vi "诊断标定3.vi"(8 "CAN端口":u16(ring), 9 "设备索引号":u16(ring), 10 "CAN卡类型":u32(ring)=21) -> ()   [LabVIEW 2013] (continued)
            n1358 = property on="配置文件版本" class="Str"("Disabled"=w1841) -> ()  [unwired: 2 in, 2 out]
            n1359 = property on="项目信息" class="Tbl (严格)"("Disabled"=w1841) -> ()  [unwired: 2 in, 2 out]
            n1360 = property on="产品编号" class="Str"("Disabled"=w1841) -> ()  [unwired: 2 in, 2 out]
            n1361 = property on="车架(牌)号" class="Str"("Disabled"=w1841) -> ()  [unwired: 2 in, 2 out]
            n1362 = Select(t=0, s=w1833, f=1) -> (s? t:f=w1832:i32)
            n1363 = property on="项目信息2" class="Clust (严格)"("DisabledEnum"=w1832) -> ()  [unwired: 2 in, 2 out]
            n1364 = property on="SOH(%)" class="DigNum (严格)"("Disabled"=w1832) -> ()  [unwired: 2 in, 2 out]
            n1365 = global read "功能码全局.vi" "主板项目信息7"() -> (w1840:bool[])
            n1366 = Index Array(array=w1840, index #1=4 ("索引"), index #2=7 ("索引")) -> (element #1=w1837:bool, element #2=w1836:bool)
            n1367 = Not(x=w1843) -> (.not. x?=w1842:bool)
          }
          frame "SOC过低(2)", "SOC过高(2)", "SOH过低(2)", "充电电流过高(2)", "单体电压过低(2)", "单体电压过高(2)", "单组电压不均衡(2)", "单组温度不均衡(2)", "二级故障阀值", "放电电流过高(2)", "极柱温度过高(2)", "内阻过大(2)", "温度过低(2)", "温度过高(2)", "整组电压不均衡(2)", "整组温度不均衡(2)", "总电压过低(2)", "总电压过高(2)" {
            w1855 = FALSE
            n1368 = property on="从板个数" class="DigNum (严格)"("NumText.BGColor"=u32 13816530) -> ()  [unwired: 2 in, 2 out]
            n1369 = Select(t=0, s=w1847, f=1) -> (s? t:f=w1846:i32)
            n1370 = property on="一级故障 2" class="Clust (严格)"("DisabledEnum"=w1846) -> ()  [unwired: 2 in, 2 out]
            n1371 = global read "功能码全局.vi" "主板故障阀值9"() -> (w1853:bool[])
            n1372 = Index Array(array=w1853, index #1=3 ("索引"), index #2=6 ("索引")) -> (element #1=w1851:bool, element #2=w1850:bool)
            n1373 = Not(x=w1855) -> (.not. x?=w1856:bool)
          }
          frame "SOC过低(3)", "SOC过高(3)", "SOH过低(3)", "充电电流过高(3)", "单体电压过低(3)", "单体电压过高(3)", "单组电压不均衡(3)", "单组温度不均衡(3)", "放电电流过高(3)", "极柱温度过高(3)", "内阻过大(3)", "三级故障阀值", "温度过低(3)", "温度过高(3)", "整组电压不均衡(3)", "整组温度不均衡(3)", "总电压过低(3)", "总电压过高(3)" {
            w1869 = FALSE
            n1374 = property on="从板个数" class="DigNum (严格)"("NumText.BGColor"=u32 13816530) -> ()  [unwired: 2 in, 2 out]
            n1375 = Select(t=0, s=w1860, f=1) -> (s? t:f=w1859:i32)
            n1376 = property on="一级故障 3" class="Clust (严格)"("DisabledEnum"=w1859) -> ()  [unwired: 2 in, 2 out]
            n1377 = global read "功能码全局.vi" "主板故障阀值9"() -> (w1866:bool[])
            n1378 = Index Array(array=w1866, index #1=4 ("索引"), index #2=7 ("索引")) -> (element #1=w1864:bool, element #2=w1863:bool)
            n1379 = Not(x=w1869) -> (.not. x?=w1868:bool)
          }
          frame "SOC过低", "SOC过高", "SOH过低", "充电电流过高", "单体电压过低", "单体电压过高", "单组电压不均衡", "单组温度不均衡", "放电电流过高", "极柱温度过高", "内阻过大", "温度过低", "温度过高", "一级故障阀值", "整组电压不均衡", "整组温度不均衡", "总电压过低", "总电压过高" {
            w1882 = FALSE
            n1380 = Select(t=0, s=w1873, f=1) -> (s? t:f=w1872:i32)
            n1381 = property on="从板个数" class="DigNum (严格)"("NumText.BGColor"=u32 13816530) -> ()  [unwired: 2 in, 2 out]
            n1382 = property on="一级故障" class="Clust (严格)"("DisabledEnum"=w1872) -> ()  [unwired: 2 in, 2 out]
            n1383 = global read "功能码全局.vi" "主板故障阀值9"() -> (w1879:bool[])
            n1384 = Index Array(array=w1879, index #1=2 ("索引"), index #2=5 ("索引")) -> (element #1=w1877:bool, element #2=w1876:bool)
            n1385 = Not(x=w1882) -> (.not. x?=w1881:bool)
          }
          frame "充电控制参数", "电流步长", "最大允许充电电流", "最大允许充电温度", "最大允许单体电压", "最大允许总电压", "最小允许充电电流", "最小允许充电温度", "最小允许单体电压" {
            w1885 = 2
            w1896 = FALSE
            n1386 = property on="从板个数" class="DigNum (严格)"("NumText.BGColor"=u32 13816530) -> ()  [unwired: 2 in, 2 out]
            n1387 = property on="风机开启温度" class="DigNum (严格)"("Disabled"=w1885) -> ()  [unwired: 2 in, 2 out]
            n1388 = property on="风机关闭温度" class="DigNum (严格)"("Disabled"=w1885) -> ()  [unwired: 2 in, 2 out]
            n1389 = property on="加热开启温度" class="DigNum (严格)"("Disabled"=w1885) -> ()  [unwired: 2 in, 2 out]
            n1390 = property on="加热关闭温度" class="DigNum (严格)"("Disabled"=w1885) -> ()  [unwired: 2 in, 2 out]
            n1391 = property on="风机开启温差" class="DigNum (严格)"("Disabled"=w1885) -> ()  [unwired: 2 in, 2 out]
            n1392 = property on="风机关闭温差" class="DigNum (严格)"("Disabled"=w1885) -> ()  [unwired: 2 in, 2 out]
            n1393 = property on="加热控制参数" class="Clust (严格)"("DisabledEnum"=w1885) -> ()  [unwired: 2 in, 2 out]
            n1394 = Select(t=0, s=w1887, f=1) -> (s? t:f=w1886:i32)
            n1395 = property on="最大允许总电压" class="DigNum (严格)"("Disabled"=w1886) -> ()  [unwired: 2 in, 2 out]
            n1396 = property on="最大允许充电温度" class="DigNum (严格)"("Disabled"=w1886) -> ()  [unwired: 2 in, 2 out]
            n1397 = property on="最小允许充电温度" class="DigNum (严格)"("Disabled"=w1886) -> ()  [unwired: 2 in, 2 out]
            n1398 = property on="电流步长" class="DigNum (严格)"("Disabled"=w1886) -> ()  [unwired: 2 in, 2 out]
            n1399 = property on="最大允许单体电压" class="DigNum (严格)"("Disabled"=w1886) -> ()  [unwired: 2 in, 2 out]
            n1400 = property on="最小允许单体电压" class="DigNum (严格)"("Disabled"=w1886) -> ()  [unwired: 2 in, 2 out]
            n1401 = property on="最大允许充电电流" class="DigNum (严格)"("Disabled"=w1886) -> ()  [unwired: 2 in, 2 out]
            n1402 = property on="最小允许充电电流" class="DigNum (严格)"("Disabled"=w1886) -> ()  [unwired: 2 in, 2 out]
            n1403 = global read "功能码全局.vi" "主板控制类信息10"() -> (w1893:bool[])
            n1404 = Index Array(array=w1893, index #1=5 ("索引"), index #2=7 ("索引")) -> (element #1=w1891:bool, element #2=w1890:bool)
            n1405 = Not(x=w1896) -> (.not. x?=w1895:bool)
          }
          frame "风机关闭温差", "风机关闭温度", "风机开启温差", "风机开启温度", "加热关闭温差", "加热关闭温度", "加热开启温度", "加热控制参数" {
            w1908 = 2
            w1910 = FALSE
            n1406 = Select(t=0, s=w1900, f=1) -> (s? t:f=w1899:i32)
            n1407 = property on="从板个数" class="DigNum (严格)"("NumText.BGColor"=u32 13816530) -> ()  [unwired: 2 in, 2 out]
            n1408 = property on="加热控制参数" class="Clust (严格)"("DisabledEnum"=w1899) -> ()  [unwired: 2 in, 2 out]
            n1409 = property on="风机开启温度" class="DigNum (严格)"("Disabled"=w1899) -> ()  [unwired: 2 in, 2 out]
            n1410 = property on="风机关闭温度" class="DigNum (严格)"("Disabled"=w1899) -> ()  [unwired: 2 in, 2 out]
            n1411 = property on="加热开启温度" class="DigNum (严格)"("Disabled"=w1899) -> ()  [unwired: 2 in, 2 out]
            n1412 = property on="加热关闭温度" class="DigNum (严格)"("Disabled"=w1899) -> ()  [unwired: 2 in, 2 out]
            n1413 = property on="风机开启温差" class="DigNum (严格)"("Disabled"=w1899) -> ()  [unwired: 2 in, 2 out]
            n1414 = property on="风机关闭温差" class="DigNum (严格)"("Disabled"=w1899) -> ()  [unwired: 2 in, 2 out]
            n1415 = property on="最大允许总电压" class="DigNum (严格)"("Disabled"=w1908) -> ()  [unwired: 2 in, 2 out]
            n1416 = property on="最大允许充电温度" class="DigNum (严格)"("Disabled"=w1908) -> ()  [unwired: 2 in, 2 out]
            n1417 = property on="最小允许充电温度" class="DigNum (严格)"("Disabled"=w1908) -> ()  [unwired: 2 in, 2 out]
            n1418 = property on="电流步长" class="DigNum (严格)"("Disabled"=w1908) -> ()  [unwired: 2 in, 2 out]
            n1419 = property on="最大允许单体电压" class="DigNum (严格)"("Disabled"=w1908) -> ()  [unwired: 2 in, 2 out]
            n1420 = property on="最小允许单体电压" class="DigNum (严格)"("Disabled"=w1908) -> ()  [unwired: 2 in, 2 out]
            n1421 = property on="最大允许充电电流" class="DigNum (严格)"("Disabled"=w1908) -> ()  [unwired: 2 in, 2 out]
            n1422 = property on="最小允许充电电流" class="DigNum (严格)"("Disabled"=w1908) -> ()  [unwired: 2 in, 2 out]
            n1423 = global read "功能码全局.vi" "主板控制类信息10"() -> (w1906:bool[])
            n1424 = Index Array(array=w1906, index #1=4 ("索引"), index #2=6 ("索引")) -> (element #1=w1904:bool, element #2=w1903:bool)
            n1425 = Not(x=w1910) -> (.not. x?=w1909:bool)
          }
          frame "电池信息" {
            w1923 = FALSE
            n1426 = Select(t=0, s=w1914, f=1) -> (s? t:f=w1913:i32)
            n1427 = property on="电池串联" class="DigNum (严格)"("Disabled"=w1913) -> ()  [unwired: 2 in, 2 out]
            n1428 = property on="电池并联" class="DigNum (严格)"("Disabled"=w1913) -> ()  [unwired: 2 in, 2 out]
            n1429 = property on="电池包额定容量" class="DigNum (严格)"("Disabled"=w1913) -> ()  [unwired: 2 in, 2 out]
            n1430 = property on="电池包额定能量(kWh)" class="DigNum (严格)"("Disabled"=w1913) -> ()  [unwired: 2 in, 2 out]
            n1431 = property on="电池包额定总电压" class="DigNum (严格)"("Disabled"=w1913) -> ()  [unwired: 2 in, 2 out]
            n1432 = property on="实际容量" class="DigNum (严格)"("Disabled"=w1913) -> ()  [unwired: 2 in, 2 out]
            n1433 = property on="电池包组号" class="Str"("Disabled"=w1913) -> ()  [unwired: 2 in, 2 out]
            n1434 = property on="电池生产日期" class="Str"("Disabled"=w1913) -> ()  [unwired: 2 in, 2 out]
            n1435 = property on="电池厂家" class="Str"("Disabled"=w1913) -> ()  [unwired: 2 in, 2 out]
            n1436 = property on="电池类型" class="Str"("Disabled"=w1913) -> ()  [unwired: 2 in, 2 out]
            n1437 = property on="累计充电总安时" class="DigNum (严格)"("Disabled"=w1913) -> ()  [unwired: 2 in, 2 out]
            n1438 = property on="累计放电总安时" class="DigNum (严格)"("Disabled"=w1913) -> ()  [unwired: 2 in, 2 out]
            n1439 = property on="电池放空次数" class="DigNum (严格)"("Disabled"=w1913) -> ()  [unwired: 2 in, 2 out]
            n1440 = property on="电池充满次数" class="DigNum (严格)"("Disabled"=w1913) -> ()  [unwired: 2 in, 2 out]
            n1441 = property on="电池充电次数" class="DigNum (严格)"("Disabled"=w1913) -> ()  [unwired: 2 in, 2 out]
            n1442 = property on="电池信息" class="Clust (严格)"("DisabledEnum"=w1913) -> ()  [unwired: 2 in, 2 out]
            n1443 = global read "功能码全局.vi" "主板版本号11"() -> (w1920:bool[])
            n1444 = property on="从板个数" class="DigNum (严格)"("NumText.BGColor"=u32 13816530) -> ()  [unwired: 2 in, 2 out]
            n1445 = Index Array(array=w1920, index #1=0 ("索引"), index #2=1 ("索引")) -> (element #1=w1918:bool, element #2=w1917:bool)
            n1446 = Not(x=w1923) -> (.not. x?=w1922:bool)
          }
          frame "电池信息1" {
            w1935 = 2
            w1937 = FALSE
            n1447 = Select(t=0, s=w1927, f=1) -> (s? t:f=w1926:i32)
            n1448 = property on="电池信息" class="Clust (严格)"("DisabledEnum"=w1926) -> ()  [unwired: 2 in, 2 out]
            n1449 = property on="电池生产日期" class="Str"("Disabled"=w1926) -> ()  [unwired: 2 in, 2 out]
            n1450 = property on="电池厂家" class="Str"("Disabled"=w1926) -> ()  [unwired: 2 in, 2 out]
            n1451 = property on="电池类型" class="Str"("Disabled"=w1926) -> ()  [unwired: 2 in, 2 out]
            n1452 = property on="电池串联" class="DigNum (严格)"("Disabled"=w1926) -> ()  [unwired: 2 in, 2 out]
            n1453 = property on="电池并联" class="DigNum (严格)"("Disabled"=w1926) -> ()  [unwired: 2 in, 2 out]
            n1454 = property on="电池包额定容量" class="DigNum (严格)"("Disabled"=w1926) -> ()  [unwired: 2 in, 2 out]
            n1455 = property on="电池包额定能量(kWh)" class="DigNum (严格)"("Disabled"=w1926) -> ()  [unwired: 2 in, 2 out]
            n1456 = property on="电池包额定总电压" class="DigNum (严格)"("Disabled"=w1926) -> ()  [unwired: 2 in, 2 out]
            n1457 = property on="实际容量" class="DigNum (严格)"("Disabled"=w1926) -> ()  [unwired: 2 in, 2 out]
            n1458 = property on="累计充电总安时" class="DigNum (严格)"("Disabled"=w1935) -> ()  [unwired: 2 in, 2 out]
            n1459 = property on="累计放电总安时" class="DigNum (严格)"("Disabled"=w1935) -> ()  [unwired: 2 in, 2 out]
            n1460 = property on="电池放空次数" class="DigNum (严格)"("Disabled"=w1935) -> ()  [unwired: 2 in, 2 out]
            n1461 = property on="电池充满次数" class="DigNum (严格)"("Disabled"=w1935) -> ()  [unwired: 2 in, 2 out]
            n1462 = property on="电池充电次数" class="DigNum (严格)"("Disabled"=w1935) -> ()  [unwired: 2 in, 2 out]
            n1463 = property on="从板个数" class="DigNum (严格)"("NumText.BGColor"=u32 13816530) -> ()  [unwired: 2 in, 2 out]
            n1464 = property on="电池包组号" class="Str"("Disabled"=w1935) -> ()  [unwired: 2 in, 2 out]
            n1465 = global read "功能码全局.vi" "主板版本号11"() -> (w1933:bool[])
            n1466 = Index Array(array=w1933, index #1=0 ("索引"), index #2=1 ("索引")) -> (element #1=w1931:bool, element #2=w1930:bool)
            n1467 = Not(x=w1937) -> (.not. x?=w1936:bool)
          }
          frame "电池包组号" {
            w1949 = 2
            w1951 = FALSE
            n1468 = property on="电池生产日期" class="Str"("Disabled"=w1949) -> ()  [unwired: 2 in, 2 out]
            n1469 = property on="电池厂家" class="Str"("Disabled"=w1949) -> ()  [unwired: 2 in, 2 out]
            n1470 = property on="电池类型" class="Str"("Disabled"=w1949) -> ()  [unwired: 2 in, 2 out]
            n1471 = property on="电池串联" class="DigNum (严格)"("Disabled"=w1949) -> ()  [unwired: 2 in, 2 out]
            n1472 = property on="电池并联" class="DigNum (严格)"("Disabled"=w1949) -> ()  [unwired: 2 in, 2 out]
            n1473 = property on="电池包额定容量" class="DigNum (严格)"("Disabled"=w1949) -> ()  [unwired: 2 in, 2 out]
            n1474 = property on="电池包额定能量(kWh)" class="DigNum (严格)"("Disabled"=w1949) -> ()  [unwired: 2 in, 2 out]
            n1475 = property on="电池包额定总电压" class="DigNum (严格)"("Disabled"=w1949) -> ()  [unwired: 2 in, 2 out]
            n1476 = property on="实际容量" class="DigNum (严格)"("Disabled"=w1949) -> ()  [unwired: 2 in, 2 out]
            n1477 = property on="从板个数" class="DigNum (严格)"("NumText.BGColor"=u32 13816530) -> ()  [unwired: 2 in, 2 out]
            n1478 = property on="累计充电总安时" class="DigNum (严格)"("Disabled"=w1949) -> ()  [unwired: 2 in, 2 out]
            n1479 = property on="累计放电总安时" class="DigNum (严格)"("Disabled"=w1949) -> ()  [unwired: 2 in, 2 out]
            n1480 = property on="电池放空次数" class="DigNum (严格)"("Disabled"=w1949) -> ()  [unwired: 2 in, 2 out]
            n1481 = property on="电池充满次数" class="DigNum (严格)"("Disabled"=w1949) -> ()  [unwired: 2 in, 2 out]
            n1482 = property on="电池充电次数" class="DigNum (严格)"("Disabled"=w1949) -> ()  [unwired: 2 in, 2 out]
            n1483 = Select(t=0, s=w1941, f=1) -> (s? t:f=w1940:i32)
            n1484 = property on="电池包组号" class="Str"("Disabled"=w1940) -> ()  [unwired: 2 in, 2 out]
            n1485 = property on="电池信息" class="Clust (严格)"("DisabledEnum"=w1940) -> ()  [unwired: 2 in, 2 out]
            n1486 = global read "功能码全局.vi" "主板版本号11"() -> (w1947:bool[])
            n1487 = Index Array(array=w1947, index #1=0 ("索引"), index #2=1 ("索引")) -> (element #1=w1945:bool, element #2=w1944:bool)
            n1488 = Not(x=w1951) -> (.not. x?=w1950:bool)
          }
          frame "充放电安时" {
            w1963 = 2
            w1965 = FALSE
            n1489 = property on="电池生产日期" class="Str"("Disabled"=w1963) -> ()  [unwired: 2 in, 2 out]
            n1490 = property on="电池厂家" class="Str"("Disabled"=w1963) -> ()  [unwired: 2 in, 2 out]
            n1491 = property on="电池类型" class="Str"("Disabled"=w1963) -> ()  [unwired: 2 in, 2 out]
            n1492 = property on="电池串联" class="DigNum (严格)"("Disabled"=w1963) -> ()  [unwired: 2 in, 2 out]
            n1493 = property on="电池并联" class="DigNum (严格)"("Disabled"=w1963) -> ()  [unwired: 2 in, 2 out]
            n1494 = property on="电池包额定容量" class="DigNum (严格)"("Disabled"=w1963) -> ()  [unwired: 2 in, 2 out]
            n1495 = property on="电池包额定能量(kWh)" class="DigNum (严格)"("Disabled"=w1963) -> ()  [unwired: 2 in, 2 out]
            n1496 = property on="电池包额定总电压" class="DigNum (严格)"("Disabled"=w1963) -> ()  [unwired: 2 in, 2 out]
            n1497 = property on="实际容量" class="DigNum (严格)"("Disabled"=w1963) -> ()  [unwired: 2 in, 2 out]
            n1498 = property on="从板个数" class="DigNum (严格)"("NumText.BGColor"=u32 13816530) -> ()  [unwired: 2 in, 2 out]
            n1499 = Select(t=0, s=w1955, f=1) -> (s? t:f=w1954:i32)
            n1500 = property on="电池放空次数" class="DigNum (严格)"("Disabled"=w1963) -> ()  [unwired: 2 in, 2 out]
            n1501 = property on="电池充满次数" class="DigNum (严格)"("Disabled"=w1963) -> ()  [unwired: 2 in, 2 out]
            n1502 = property on="电池充电次数" class="DigNum (严格)"("Disabled"=w1963) -> ()  [unwired: 2 in, 2 out]
            n1503 = property on="电池包组号" class="Str"("Disabled"=w1963) -> ()  [unwired: 2 in, 2 out]
            n1504 = property on="累计充电总安时" class="DigNum (严格)"("Disabled"=w1954) -> ()  [unwired: 2 in, 2 out]
            n1505 = property on="累计放电总安时" class="DigNum (严格)"("Disabled"=w1954) -> ()  [unwired: 2 in, 2 out]
            n1506 = property on="电池信息" class="Clust (严格)"("DisabledEnum"=w1954) -> ()  [unwired: 2 in, 2 out]
            n1507 = global read "功能码全局.vi" "主板版本号11"() -> (w1961:bool[])
            n1508 = Index Array(array=w1961, index #1=0 ("索引"), index #2=1 ("索引")) -> (element #1=w1959:bool, element #2=w1958:bool)
            n1509 = Not(x=w1965) -> (.not. x?=w1964:bool)
          }
          frame "电池充放电次数" {
            w1977 = 2
            w1979 = FALSE
            n1510 = property on="从板个数" class="DigNum (严格)"("NumText.BGColor"=u32 13816530) -> ()  [unwired: 2 in, 2 out]
            n1511 = property on="电池生产日期" class="Str"("Disabled"=w1977) -> ()  [unwired: 2 in, 2 out]
            n1512 = property on="电池厂家" class="Str"("Disabled"=w1977) -> ()  [unwired: 2 in, 2 out]
            n1513 = property on="电池类型" class="Str"("Disabled"=w1977) -> ()  [unwired: 2 in, 2 out]
            n1514 = property on="电池串联" class="DigNum (严格)"("Disabled"=w1977) -> ()  [unwired: 2 in, 2 out]
            n1515 = property on="电池并联" class="DigNum (严格)"("Disabled"=w1977) -> ()  [unwired: 2 in, 2 out]
            n1516 = property on="电池包额定容量" class="DigNum (严格)"("Disabled"=w1977) -> ()  [unwired: 2 in, 2 out]
            n1517 = property on="电池包额定能量(kWh)" class="DigNum (严格)"("Disabled"=w1977) -> ()  [unwired: 2 in, 2 out]
            n1518 = property on="电池包额定总电压" class="DigNum (严格)"("Disabled"=w1977) -> ()  [unwired: 2 in, 2 out]
            n1519 = property on="实际容量" class="DigNum (严格)"("Disabled"=w1977) -> ()  [unwired: 2 in, 2 out]
            n1520 = Select(t=0, s=w1969, f=1) -> (s? t:f=w1968:i32)
            n1521 = property on="电池放空次数" class="DigNum (严格)"("Disabled"=w1968) -> ()  [unwired: 2 in, 2 out]
            n1522 = property on="电池充满次数" class="DigNum (严格)"("Disabled"=w1968) -> ()  [unwired: 2 in, 2 out]
            n1523 = property on="电池充电次数" class="DigNum (严格)"("Disabled"=w1968) -> ()  [unwired: 2 in, 2 out]
            n1524 = property on="累计充电总安时" class="DigNum (严格)"("Disabled"=w1977) -> ()  [unwired: 2 in, 2 out]
            n1525 = property on="累计放电总安时" class="DigNum (严格)"("Disabled"=w1977) -> ()  [unwired: 2 in, 2 out]
            n1526 = property on="电池信息" class="Clust (严格)"("DisabledEnum"=w1968) -> ()  [unwired: 2 in, 2 out]
            n1527 = property on="电池包组号" class="Str"("Disabled"=w1977) -> ()  [unwired: 2 in, 2 out]
            n1528 = global read "功能码全局.vi" "主板版本号11"() -> (w1975:bool[])
            n1529 = Index Array(array=w1975, index #1=0 ("索引"), index #2=1 ("索引")) -> (element #1=w1973:bool, element #2=w1972:bool)
            n1530 = Not(x=w1979) -> (.not. x?=w1978:bool)
          }
          frame "假", Default {
            w1984 = FALSE
            n1531 = Not(x=w1984) -> (.not. x?=w1983:bool)
          }
        }
        n1532 = property on="单个读取" class="Bool (严格)"("Visible"=w1452) -> ()  [unwired: 2 in, 2 out]
        n1533 = property on="单个写入" class="Bool (严格)"("Visible"=w1451) -> ()  [unwired: 2 in, 2 out]
        n1534 = local write "1"(w1459) -> ()
        n1535 = local write "1 2"(w1458) -> ()
        n1536 = local write "1 3"(w1457) -> ()
        n1537 = local write "1 4"(w1456) -> ()
        n1538 = local write "1 5"(w1455) -> ()
        n1539 = local write "1 11"(w1454) -> ()
        n1540 = local write "主板2"(w1460) -> ()
      }
      event "从板选项": Mouse Down {
        n1541 = event-data() -> ("CtlRef"=w1999:refnum<vi>)  [unwired: 8 out]
        n1542 = property class="Tree (严格)"(reference=w1999) -> ("Value"=w1998:string)  [unwired: 1 in, 2 out]
        n1543 = global read "功能码全局.vi" "主板监控2"() -> (w1989:bool[])
        n1544 = Index Array(array=w1989, index=6 ("索引")) -> (element=w1987:bool)
        n1545 = case shown="\"二维码\"" w1998 {
          tunnel: [T19."从板信息" ("等级 2") T19."从板信息" ("等级 2") T19."从板信息" ("等级 2") T19."从板信息" ("等级 2") T19."从板信息" ("等级 2") T19."从板信息" ("等级 2") T19."从板信息" ("等级 2") T19."从板信息" ("等级 2") T19."一级故障阀值" ("等级 2") T19."二级故障阀值" ("等级 2") T19."三级故障阀值" ("等级 2") T19."快换参数" ("等级 2") T19."快换参数" ("等级 2") T19."快换参数" ("等级 2") T19."快换参数" ("等级 2") T19."快换参数" ("等级 2") T19."快换参数" ("等级 2") T19."快换参数" ("等级 2") T19."快换参数" ("等级 2") T14."均衡参数" ("等级 2") T14."均衡参数" ("等级 2") T14."均衡参数" ("等级 2") T19."从板信息" ("等级 2")] -> w1997
          tunnel: [w2010 w2020 w2030 w2044 w2059 w2094 w2131 w2168 w2192 w2205 w2218 w2231 w2257 w2271 w2287 w2304 w2321 w2339 w2358 w2375 w2388 w2402 w2417] -> w1996
          tunnel: [w2002 w2012 w2022 w2032 w2046 w2081 w2118 w2155 w2203 w2205 w2218 w2231 w2257 w2271 w2287 w2304 w2321 w2339 w2358 w2375 w2388 w2402 w2416] -> w1995
          tunnel: [w2002 w2012 w2022 w2032 w2046 w2081 w2118 w2155 w2192 w2216 w2218 w2231 w2257 w2271 w2287 w2304 w2321 w2339 w2358 w2375 w2388 w2402 w2416] -> w1994
          tunnel: [w2002 w2012 w2022 w2032 w2046 w2081 w2118 w2155 w2192 w2205 w2229 w2231 w2257 w2271 w2287 w2304 w2321 w2339 w2358 w2375 w2388 w2402 w2416] -> w1993
          tunnel: [w2002 w2012 w2022 w2032 w2046 w2081 w2118 w2155 w2192 w2205 w2218 w2255 w2269 w2285 w2302 w2319 w2337 w2356 w2373 w2375 w2388 w2402 w2416] -> w1992
          tunnel: [w2007 w2017 w2023 w2039 w2053 w2088 w2125 w2162 w2199 w2212 w2225 w2240 w2262 w2277 w2291 w2309 w2324 w2344 w2362 w2378 w2392 w2407 w2416] -> w1991
          tunnel: [w2004 w2014 w2023 w2038 w2052 w2087 w2124 w2161 w2198 w2211 w2224 w2232 w2261 w2276 w2290 w2310 w2325 w2343 w2361 w2377 w2391 w2406 w2416] -> w1990
          tunnel: w1987 -> [_ _ w2027 w2035 w2049 w2084 w2121 w2158 w2194 w2208 w2221 w2252 w2265 w2280 w2295 w2313 w2329 w2347 w2366 w2381 w2395 w2409 _]
          tunnel: [w2002 w2012 w2022 w2032 w2046 w2081 w2118 w2155 w2192 w2205 w2218 w2231 w2257 w2271 w2287 w2304 w2321 w2339 w2358 w2376 w2389 w2403 w2416] -> w1986
          frame "从板号" {
            w2009 = 2
            w2002 = FALSE ("1 6")
            n1546 = property on="项目信息 2" class="Tbl (严格)"("Disabled"=w2009) -> ()  [unwired: 2 in, 2 out]
            n1547 = property on="加热控制参数" class="Clust (严格)"("Disabled"=w2009) -> ()  [unwired: 2 in, 2 out]
            n1548 = property on="从板号" class="DigNum (严格)"("NumText.BGColor"=u32 6618880) -> ()  [unwired: 2 in, 2 out]
            n1549 = global read "功能码全局.vi" "16"() -> (w2006:bool[])
            n1550 = Index Array(array=w2006, index #1=4 ("索引"), index #2=6 ("索引")) -> (element #1=w2007:bool, element #2=w2004:bool)
            n1551 = Not(x=w2002) -> (.not. x?=w2010:bool)
          }
          frame "二维码" {
            w2019 = 2
            w2012 = FALSE ("1 6")
            n1552 = property on="项目信息 2" class="Tbl (严格)"("Disabled"=w2019) -> ()  [unwired: 2 in, 2 out]
            n1553 = property on="加热控制参数" class="Clust (严格)"("Disabled"=w2019) -> ()  [unwired: 2 in, 2 out]
            n1554 = property on="从板号" class="DigNum (严格)"("NumText.BGColor"=u32 6618880) -> ()  [unwired: 2 in, 2 out]
            n1555 = global read "功能码全局.vi" "16"() -> (w2016:bool[])
            n1556 = Index Array(array=w2016, index #1=4 ("索引"), index #2=6 ("索引")) -> (element #1=w2017:bool, element #2=w2014:bool)
            n1557 = Not(x=w2012) -> (.not. x?=w2020:bool)
          }
          frame "从板信息" {
            w2022 = FALSE ("1 6")
            n1558 = Select(t=0, s=w2027, f=1) -> (s? t:f=w2026:i32)
            n1559 = property on="从板号" class="DigNum (严格)"("NumText.BGColor"=u32 16777215) -> ()  [unwired: 2 in, 2 out]
            n1560 = property on="项目信息 2" class="Tbl (严格)"("Disabled"=w2026) -> ()  [unwired: 2 in, 2 out]
            n1561 = property on="加热控制参数" class="Clust (严格)"("Disabled"=w2026) -> ()  [unwired: 2 in, 2 out]
            n1562 = Not(x=w2022) -> (.not. x?=w2030:bool)
            n1563 = local read "从板项目信息"() -> (w2024:bool)
            n1564 = Not(x=w2024) -> (.not. x?=w2023:bool)
          }
          frame "风机关闭温差", "风机关闭温度", "风机开启温差", "风机开启温度", "加热关闭温差", "加热关闭温度", "加热开启温度", "加热控制参数" {
            w2032 = FALSE ("1 6")
            n1565 = property on="从板号" class="DigNum (严格)"("NumText.BGColor"=u32 16777215) -> ()  [unwired: 2 in, 2 out]
            n1566 = Select(t=0, s=w2035, f=1) -> (s? t:f=w2034:i32)
            n1567 = property on="项目信息 2" class="Tbl (严格)"("Disabled"=2) -> ()  [unwired: 2 in, 2 out]
            n1568 = property on="加热控制参数" class="Clust (严格)"("Disabled"=w2034) -> ()  [unwired: 2 in, 2 out]
            n1569 = global read "功能码全局.vi" "16"() -> (w2041:bool[])
            n1570 = Index Array(array=w2041, index #1=5 ("索引"), index #2=7 ("索引")) -> (element #1=w2039:bool, element #2=w2038:bool)
            n1571 = Not(x=w2032) -> (.not. x?=w2044:bool)
          }
          frame "电压个数" {
            w2046 = FALSE ("1 6")
            n1572 = property on="从板号" class="DigNum (严格)"("NumText.BGColor"=u32 16777215) -> ()  [unwired: 2 in, 2 out]
            n1573 = control-ref of="项目信息 2"() -> (w2057:refnum<vi>)
            n1574 = stacked-sequence {
              tunnel: w2057 -> [w2064 w2066 w2075]
              frame #0 {
                n1575 = Bundle(0, 0) -> (w2063:cluster{i32, i32})  [unwired: 1 out]
                n1576 = property class="Tbl (严格)"(reference=w2064, "Index Values"=w2063) -> ()  [unwired: 1 in, 2 out]
              }
              frame #1 {
                n1577 = for {
                  N: 40 -> [_]
                  tunnel: w2066 -> [w2073]
                  i -> [w2068]
                  n1578 = Compound Arithmetic op=ADD(0 ("值"), w2068) -> (w2070:i32)
                  n1579 = Bundle(w2070, 0) -> (w2072:cluster{i32, i32})  [unwired: 1 out]
                  n1580 = property class="Tbl (严格)"(reference=w2073, "Active Cell"=w2072, "Cell BG Color"=u32 16448250) -> ()  [unwired: 1 in, 2 out]
                }
              }
              frame #2 {
                n1581 = for {
                  N: 1 -> [_]
                  tunnel: w2075 -> [w2080]
                  i -> [w2076]
                  n1582 = Bundle(w2076, 0) -> (w2079:cluster{i32, i32})  [unwired: 1 out]
                  n1583 = property class="Tbl (严格)"(reference=w2080, "Active Cell"=w2079, "Cell BG Color"=u32 6618880) -> ()  [unwired: 1 in, 2 out]
                }
              }
            }
            n1584 = Select(t=0, s=w2049, f=1) -> (s? t:f=w2048:i32)
            n1585 = property on="项目信息 2" class="Tbl (严格)"("Disabled"=w2048) -> ()  [unwired: 2 in, 2 out]
            n1586 = property on="加热控制参数" class="Clust (严格)"("Disabled"=2) -> ()  [unwired: 2 in, 2 out]
            n1587 = global read "功能码全局.vi" "15"() -> (w2055:bool[])
            n1588 = Index Array(array=w2055, index #1=0 ("索引"), index #2=4 ("索引")) -> (element #1=w2053:bool, element #2=w2052:bool)
            n1589 = Not(x=w2046) -> (.not. x?=w2059:bool)
          }
          frame "通道电压节数" {
            w2081 = FALSE ("1 6")
            n1590 = property on="从板号" class="DigNum (严格)"("NumText.BGColor"=u32 16777215) -> ()  [unwired: 2 in, 2 out]
            n1591 = control-ref of="项目信息 2"() -> (w2092:refnum<vi>)
            n1592 = stacked-sequence {
              tunnel: w2092 -> [w2099 w2101 w2110]
              frame #0 {
                n1593 = Bundle(22, 0) -> (w2098:cluster{i32, i32})  [unwired: 1 out]
                n1594 = property class="Tbl (严格)"(reference=w2099, "Index Values"=w2098) -> ()  [unwired: 1 in, 2 out]
              }
              frame #1 {
                n1595 = for {
                  N: 40 -> [_]
                  tunnel: w2101 -> [w2108]
                  i -> [w2103]
                  n1596 = Compound Arithmetic op=ADD(0 ("值"), w2103) -> (w2105:i32)
                  n1597 = Bundle(w2105, 0) -> (w2107:cluster{i32, i32})  [unwired: 1 out]
                  n1598 = property class="Tbl (严格)"(reference=w2108, "Active Cell"=w2107, "Cell BG Color"=u32 16448250) -> ()  [unwired: 1 in, 2 out]
                }
              }
              frame #2 {
                n1599 = for {
                  N: 5 -> [_]
                  tunnel: w2110 -> [w2117]
                  i -> [w2113]
                  n1600 = Add(x=22, y=w2113) -> (x+y=w2112:i32)
                  n1601 = Bundle(w2112, 0) -> (w2116:cluster{i32, i32})  [unwired: 1 out]
                  n1602 = property class="Tbl (严格)"(reference=w2117, "Active Cell"=w2116, "Cell BG Color"=u32 6618880) -> ()  [unwired: 1 in, 2 out]
                }
              }
            }
            n1603 = Select(t=0, s=w2084, f=1) -> (s? t:f=w2083:i32)
            n1604 = property on="项目信息 2" class="Tbl (严格)"("Disabled"=w2083) -> ()  [unwired: 2 in, 2 out]
            n1605 = property on="加热控制参数" class="Clust (严格)"("Disabled"=2) -> ()  [unwired: 2 in, 2 out]
            n1606 = global read "功能码全局.vi" "15"() -> (w2090:bool[])
            n1607 = Index Array(array=w2090, index #1=1 ("索引"), index #2=5 ("索引")) -> (element #1=w2088:bool, element #2=w2087:bool)
            n1608 = Not(x=w2081) -> (.not. x?=w2094:bool)
          }
          frame "保险位置" {
            w2118 = FALSE ("1 6")
            n1609 = control-ref of="项目信息 2"() -> (w2129:refnum<vi>)
            n1610 = stacked-sequence {
              tunnel: w2129 -> [w2136 w2138 w2147]
              frame #0 {
                n1611 = Bundle(0, 0) -> (w2135:cluster{i32, i32})  [unwired: 1 out]
                n1612 = property class="Tbl (严格)"(reference=w2136, "Index Values"=w2135) -> ()  [unwired: 1 in, 2 out]
              }
              frame #1 {
                n1613 = for {
                  N: 40 -> [_]
                  tunnel: w2138 -> [w2145]
                  i -> [w2141]
                  n1614 = Add(x=2, y=w2141) -> (x+y=w2140:i32)
                  n1615 = Bundle(w2140, 0) -> (w2144:cluster{i32, i32})  [unwired: 1 out]
                  n1616 = property class="Tbl (严格)"(reference=w2145, "Active Cell"=w2144, "Cell BG Color"=u32 16448250) -> ()  [unwired: 1 in, 2 out]
                }
              }
              frame #2 {
                n1617 = for {
                  N: 20 -> [_]
                  tunnel: w2147 -> [w2154]
                  i -> [w2150]
                  n1618 = Add(x=2, y=w2150) -> (x+y=w2149:i32)
                  n1619 = Bundle(w2149, 0) -> (w2153:cluster{i32, i32})  [unwired: 1 out]
                  n1620 = property class="Tbl (严格)"(reference=w2154, "Active Cell"=w2153, "Cell BG Color"=u32 6618880) -> ()  [unwired: 1 in, 2 out]
                }
              }
            }
            n1621 = property on="从板号" class="DigNum (严格)"("NumText.BGColor"=u32 16777215) -> ()  [unwired: 2 in, 2 out]
            n1622 = Select(t=0, s=w2121, f=1) -> (s? t:f=w2120:i32)
            n1623 = property on="项目信息 2" class="Tbl (严格)"("Disabled"=w2120) -> ()  [unwired: 2 in, 2 out]
            n1624 = property on="加热控制参数" class="Clust (严格)"("Disabled"=2) -> ()  [unwired: 2 in, 2 out]
            n1625 = global read "功能码全局.vi" "15"() -> (w2127:bool[])
            n1626 = Index Array(array=w2127, index #1=2 ("索引"), index #2=6 ("索引")) -> (element #1=w2125:bool, element #2=w2124:bool)
            n1627 = Not(x=w2118) -> (.not. x?=w2131:bool)
          }
          frame "温度个数" {
            w2155 = FALSE ("1 6")
            n1628 = control-ref of="项目信息 2"() -> (w2166:refnum<vi>)
            n1629 = stacked-sequence {
              tunnel: w2166 -> [w2173 w2174 w2184]
              frame #0 {
                n1630 = Bundle(0, 0) -> (w2172:cluster{i32, i32})  [unwired: 1 out]
                n1631 = property class="Tbl (严格)"(reference=w2173, "Index Values"=w2172) -> ()  [unwired: 1 in, 2 out]
              }
              frame #1 {
                n1632 = for {
                  N: 40 -> [_]
                  tunnel: w2174 -> [w2182]
                  i -> [w2177]
                  n1633 = Compound Arithmetic op=ADD(0 ("值"), w2177) -> (w2179:i32)
                  n1634 = Bundle(w2179, 0) -> (w2181:cluster{i32, i32})  [unwired: 1 out]
                  n1635 = property class="Tbl (严格)"(reference=w2182, "Active Cell"=w2181, "Cell BG Color"=u32 16448250) -> ()  [unwired: 1 in, 2 out]
                }
              }
              frame #2 {
                n1636 = for {
                  N: 1 -> [_]
                  tunnel: w2184 -> [w2191]
                  i -> [w2187]
                  n1637 = Add(x=1, y=w2187) -> (x+y=w2186:i32)
                  n1638 = Bundle(w2186, 0) -> (w2190:cluster{i32, i32})  [unwired: 1 out]
                  n1639 = property class="Tbl (严格)"(reference=w2191, "Active Cell"=w2190, "Cell BG Color"=u32 6618880) -> ()  [unwired: 1 in, 2 out]
                }
              }
            }
            n1640 = Select(t=0, s=w2158, f=1) -> (s? t:f=w2157:i32)
            n1641 = property on="项目信息 2" class="Tbl (严格)"("Disabled"=w2157) -> ()  [unwired: 2 in, 2 out]
            n1642 = property on="加热控制参数" class="Clust (严格)"("Disabled"=2) -> ()  [unwired: 2 in, 2 out]
            n1643 = property on="从板号" class="DigNum (严格)"("NumText.BGColor"=u32 16777215) -> ()  [unwired: 2 in, 2 out]
            n1644 = global read "功能码全局.vi" "15"() -> (w2164:bool[])
            n1645 = Index Array(array=w2164, index #1=3 ("索引"), index #2=7 ("索引")) -> (element #1=w2162:bool, element #2=w2161:bool)
            n1646 = Not(x=w2155) -> (.not. x?=w2168:bool)
          }
          frame "SOC过低", "电压不均衡", "电压过低", "电压过高", "温度不均衡", "温度过低", "温度过高", "一级故障阀值" {
            w2192 = FALSE ("1 6")
            n1647 = property on="从板号" class="DigNum (严格)"("NumText.BGColor"=u32 16777215) -> ()  [unwired: 2 in, 2 out]
            n1648 = Select(t=0, s=w2194, f=1) -> (s? t:f=w2195:i32)
            n1649 = property on="一级故障 6" class="Clust (严格)"("DisabledEnum"=w2195) -> ()  [unwired: 2 in, 2 out]
            n1650 = global read "功能码全局.vi" "18"() -> (w2201:bool[])
            n1651 = Index Array(array=w2201, index #1=2 ("索引"), index #2=5 ("索引")) -> (element #1=w2199:bool, element #2=w2198:bool)
            n1652 = Not(x=w2192) -> (.not. x?=w2203:bool)
          }
          frame "SOC过低(2)", "电压不均衡(2)", "电压过低(2)", "电压过高(2)", "二级故障阀值", "温度不均衡(2)", "温度过低(2)", "温度过高(2)" {
            w2205 = FALSE ("1 6")
            n1653 = property on="从板号" class="DigNum (严格)"("NumText.BGColor"=u32 16777215) -> ()  [unwired: 2 in, 2 out]
            n1654 = Select(t=0, s=w2208, f=1) -> (s? t:f=w2207:i32)
            n1655 = property on="一级故障 7" class="Clust (严格)"("DisabledEnum"=w2207) -> ()  [unwired: 2 in, 2 out]
            n1656 = global read "功能码全局.vi" "18"() -> (w2214:bool[])
            n1657 = Index Array(array=w2214, index #1=3 ("索引"), index #2=6 ("索引")) -> (element #1=w2212:bool, element #2=w2211:bool)
            n1658 = Not(x=w2205) -> (.not. x?=w2216:bool)
          }
          frame "SOC过低(3)", "电压不均衡(3)", "电压过低(3)", "电压过高(3)", "三级故障阀值", "温度不均衡(3)", "温度过低(3)", "温度过高(3)" {
            w2218 = FALSE ("1 6")
            n1659 = property on="从板号" class="DigNum (严格)"("NumText.BGColor"=u32 16777215) -> ()  [unwired: 2 in, 2 out]
            n1660 = Select(t=0, s=w2221, f=1) -> (s? t:f=w2220:i32)
            n1661 = property on="一级故障 8" class="Clust (严格)"("DisabledEnum"=w2220) -> ()  [unwired: 2 in, 2 out]
            n1662 = global read "功能码全局.vi" "18"() -> (w2227:bool[])
            n1663 = Index Array(array=w2227, index #1=4 ("索引"), index #2=7 ("索引")) -> (element #1=w2225:bool, element #2=w2224:bool)
            n1664 = Not(x=w2218) -> (.not. x?=w2229:bool)
          }
          frame "快换参数" {
            w2231 = FALSE ("1 6")
            n1665 = Select(t=0, s=w2252, f=1) -> (s? t:f=w2251:i32)
            n1666 = property on="电池组信息" class="Clust (严格)"("Disabled"=w2251) -> ()  [unwired: 2 in, 2 out]
            n1667 = property on="从板号" class="DigNum (严格)"("NumText.BGColor"=u32 16777215) -> ()  [unwired: 2 in, 2 out]
            n1668 = global read "功能码全局.vi" "24"() -> (w2248:bool[])
            n1669 = global read "功能码全局.vi" "23"() -> (w2249:bool[])
            n1670 = Index Array(array=w2248) -> (element #3=w2238:bool, element #4=w2237:bool, element #5=w2236:bool, element #6=w2235:bool, element #7=w2234:bool, element #8=w2233:bool)  [unwired: 8 in, 2 out]
            n1671 = Index Array(array=w2249) -> (element #3=w2247:bool, element #4=w2246:bool, element #5=w2245:bool, element #6=w2244:bool, element #7=w2243:bool, element #8=w2242:bool)  [unwired: 8 in, 2 out]
            n1672 = Build Array(w2238, w2237, w2236, w2235, w2234, w2233) -> (w2239:bool[])
            n1673 = Build Array(w2247, w2246, w2245, w2244, w2243, w2242) -> (w2241:bool[])
            n1674 = And Array Elements(Boolean array=w2239) -> (logical AND=w2232:bool)
            n1675 = And Array Elements(Boolean array=w2241) -> (logical AND=w2240:bool)
            n1676 = Not(x=w2231) -> (.not. x?=w2255:bool)
          }
          frame "电池包信息1" {
            w2260 = 2
            w2268 = 2
            w2259 = 2
            w2257 = FALSE ("1 6")
            n1677 = Select(t=0, s=w2265, f=1) -> (s? t:f=w2258:i32)
            n1678 = property on="串联数" class="DigNum (严格)"("Disabled"=w2258) -> ()  [unwired: 2 in, 2 out]
            n1679 = property on="并联数" class="DigNum (严格)"("Disabled"=w2258) -> ()  [unwired: 2 in, 2 out]
            n1680 = property on="电池厂家" class="DigNum (严格)"("Disabled"=w2258) -> ()  [unwired: 2 in, 2 out]
            n1681 = property on="电池类型" class="DigNum (严格)"("Disabled"=w2258) -> ()  [unwired: 2 in, 2 out]
            n1682 = property on="额定能量" class="DigNum (严格)"("Disabled"=w2258) -> ()  [unwired: 2 in, 2 out]
            n1683 = property on="额定容量" class="DigNum (严格)"("Disabled"=w2258) -> ()  [unwired: 2 in, 2 out]
            n1684 = property on="实际容量" class="DigNum (严格)"("Disabled"=w2258) -> ()  [unwired: 2 in, 2 out]
            n1685 = property on="电池组信息" class="Clust (严格)"("Disabled"=w2258) -> ()  [unwired: 2 in, 2 out]
            n1686 = property on="生产日期" class="Str"("DisabledEnum"=w2258) -> ()  [unwired: 2 in, 2 out]
            n1687 = property on="车牌号" class="Str"("DisabledEnum"=w2259) -> ()  [unwired: 2 in, 2 out]
            n1688 = property on="产权标识" class="DigNum (严格)"("Disabled"=w2258) -> ()  [unwired: 2 in, 2 out]
            n1689 = property on="应用车型" class="DigNum (严格)"("Disabled"=w2258) -> ()  [unwired: 2 in, 2 out]
            n1690 = property on="额定总压" class="DigNum (严格)"("Disabled"=w2258) -> ()  [unwired: 2 in, 2 out]
            n1691 = property on="电池包序号" class="DigNum (严格)"("DisabledEnum"=w2258) -> ()  [unwired: 2 in, 2 out]
            n1692 = property on="电池包组号" class="DigNum (严格)"("DisabledEnum"=w2259) -> ()  [unwired: 2 in, 2 out]
            n1693 = property on="最大允许单体电压" class="DigNum (严格)"("Disabled"=w2268) -> ()  [unwired: 2 in, 2 out]
            n1694 = property on="最大允许总电压" class="DigNum (严格)"("Disabled"=w2268) -> ()  [unwired: 2 in, 2 out]
            n1695 = property on="最大允许温度" class="DigNum (严格)"("Disabled"=w2268) -> ()  [unwired: 2 in, 2 out]
            n1696 = property on="最小允许温度" class="DigNum (严格)"("Disabled"=w2268) -> ()  [unwired: 2 in, 2 out]
            n1697 = property on="最大允许充电电流" class="DigNum (严格)"("Disabled"=w2268) -> ()  [unwired: 2 in, 2 out]
            n1698 = property on="最小允许充电电流" class="DigNum (严格)"("Disabled"=w2268) -> ()  [unwired: 2 in, 2 out]
            n1699 = property on="最小允许单体电压" class="DigNum (严格)"("Disabled"=w2268) -> ()  [unwired: 2 in, 2 out]
            n1700 = property on="电流步长" class="DigNum (严格)"("Disabled"=w2268) -> ()  [unwired: 2 in, 2 out]
            n1701 = property on="SOC" class="DigNum (严格)"("Disabled"=w2268) -> ()  [unwired: 2 in, 2 out]
            n1702 = property on="充电总安时" class="DigNum (严格)"("Disabled"=w2268) -> ()  [unwired: 2 in, 2 out]
            n1703 = property on="放电总安时" class="DigNum (严格)"("Disabled"=w2268) -> ()  [unwired: 2 in, 2 out]
            n1704 = property on="放空次数" class="DigNum (严格)"("DisabledEnum"=w2260) -> ()  [unwired: 2 in, 2 out]
            n1705 = property on="充满次数" class="DigNum (严格)"("DisabledEnum"=w2260) -> ()  [unwired: 2 in, 2 out]
            n1706 = property on="充电次数" class="DigNum (严格)"("DisabledEnum"=w2260) -> ()  [unwired: 2 in, 2 out]
            n1707 = global read "功能码全局.vi" "24"() -> (w2263:bool[])
            n1708 = global read "功能码全局.vi" "23"() -> (w2264:bool[])
            n1709 = Index Array(array=w2263) -> (element #3=w2261:bool)  [unwired: 8 in, 7 out]
            n1710 = Index Array(array=w2264) -> (element #3=w2262:bool)  [unwired: 8 in, 7 out]
            n1711 = Not(x=w2257) -> (.not. x?=w2269:bool)
          }
          frame "电池包组号" {
            w2274 = 2
            w2273 = 2
            w2283 = 2
            w2275 = 2
            w2284 = 2
            w2271 = FALSE ("1 6")
            n1712 = property on="串联数" class="DigNum (严格)"("Disabled"=w2284) -> ()  [unwired: 2 in, 2 out]
            n1713 = property on="并联数" class="DigNum (严格)"("Disabled"=w2284) -> ()  [unwired: 2 in, 2 out]
            n1714 = property on="电池厂家" class="DigNum (严格)"("Disabled"=w2284) -> ()  [unwired: 2 in, 2 out]
            n1715 = property on="电池类型" class="DigNum (严格)"("Disabled"=w2284) -> ()  [unwired: 2 in, 2 out]
            n1716 = property on="额定能量" class="DigNum (严格)"("Disabled"=w2284) -> ()  [unwired: 2 in, 2 out]
            n1717 = property on="额定容量" class="DigNum (严格)"("Disabled"=w2284) -> ()  [unwired: 2 in, 2 out]
            n1718 = property on="实际容量" class="DigNum (严格)"("Disabled"=w2284) -> ()  [unwired: 2 in, 2 out]
            n1719 = Select(t=0, s=w2280, f=1) -> (s? t:f=w2272:i32)
            n1720 = property on="生产日期" class="Str"("DisabledEnum"=w2274) -> ()  [unwired: 2 in, 2 out]
            n1721 = property on="电池包序号" class="DigNum (严格)"("DisabledEnum"=w2274) -> ()  [unwired: 2 in, 2 out]
            n1722 = property on="车牌号" class="Str"("DisabledEnum"=w2274) -> ()  [unwired: 2 in, 2 out]
            n1723 = property on="电池包组号" class="DigNum (严格)"("DisabledEnum"=w2272) -> ()  [unwired: 2 in, 2 out]
            n1724 = property on="电池组信息" class="Clust (严格)"("Disabled"=w2272) -> ()  [unwired: 2 in, 2 out]
            n1725 = property on="产权标识" class="DigNum (严格)"("Disabled"=w2275) -> ()  [unwired: 2 in, 2 out]
            n1726 = property on="应用车型" class="DigNum (严格)"("Disabled"=w2275) -> ()  [unwired: 2 in, 2 out]
            n1727 = property on="额定总压" class="DigNum (严格)"("Disabled"=w2275) -> ()  [unwired: 2 in, 2 out]
            n1728 = property on="放空次数" class="DigNum (严格)"("DisabledEnum"=w2273) -> ()  [unwired: 2 in, 2 out]
            n1729 = property on="充满次数" class="DigNum (严格)"("DisabledEnum"=w2273) -> ()  [unwired: 2 in, 2 out]
            n1730 = property on="充电次数" class="DigNum (严格)"("DisabledEnum"=w2273) -> ()  [unwired: 2 in, 2 out]
            n1731 = property on="最大允许单体电压" class="DigNum (严格)"("Disabled"=w2283) -> ()  [unwired: 2 in, 2 out]
            n1732 = property on="最大允许总电压" class="DigNum (严格)"("Disabled"=w2283) -> ()  [unwired: 2 in, 2 out]
            n1733 = property on="最大允许温度" class="DigNum (严格)"("Disabled"=w2283) -> ()  [unwired: 2 in, 2 out]
            n1734 = property on="最小允许温度" class="DigNum (严格)"("Disabled"=w2283) -> ()  [unwired: 2 in, 2 out]
            n1735 = property on="最大允许充电电流" class="DigNum (严格)"("Disabled"=w2283) -> ()  [unwired: 2 in, 2 out]
            n1736 = property on="最小允许充电电流" class="DigNum (严格)"("Disabled"=w2283) -> ()  [unwired: 2 in, 2 out]
            n1737 = property on="最小允许单体电压" class="DigNum (严格)"("Disabled"=w2283) -> ()  [unwired: 2 in, 2 out]
            n1738 = property on="电流步长" class="DigNum (严格)"("Disabled"=w2283) -> ()  [unwired: 2 in, 2 out]
            n1739 = property on="SOC" class="DigNum (严格)"("Disabled"=w2283) -> ()  [unwired: 2 in, 2 out]
            n1740 = property on="充电总安时" class="DigNum (严格)"("Disabled"=w2283) -> ()  [unwired: 2 in, 2 out]
            n1741 = property on="放电总安时" class="DigNum (严格)"("Disabled"=w2283) -> ()  [unwired: 2 in, 2 out]
            n1742 = global read "功能码全局.vi" "24"() -> (w2278:bool[])
            n1743 = global read "功能码全局.vi" "23"() -> (w2279:bool[])
            n1744 = Index Array(array=w2278) -> (element #3=w2276:bool)  [unwired: 8 in, 7 out]
            n1745 = Index Array(array=w2279) -> (element #3=w2277:bool)  [unwired: 8 in, 7 out]
            n1746 = Not(x=w2271) -> (.not. x?=w2285:bool)
          }
          frame "充放电安时" {
            w2289 = 2
            w2288 = 2
            w2298 = 2
            w2299 = 2
            w2301 = 2
            w2287 = FALSE ("1 6")
            n1747 = property on="串联数" class="DigNum (严格)"("Disabled"=w2301) -> ()  [unwired: 2 in, 2 out]
            n1748 = property on="并联数" class="DigNum (严格)"("Disabled"=w2301) -> ()  [unwired: 2 in, 2 out]
            n1749 = property on="电池厂家" class="DigNum (严格)"("Disabled"=w2301) -> ()  [unwired: 2 in, 2 out]
            n1750 = property on="电池类型" class="DigNum (严格)"("Disabled"=w2301) -> ()  [unwired: 2 in, 2 out]
            n1751 = property on="额定能量" class="DigNum (严格)"("Disabled"=w2301) -> ()  [unwired: 2 in, 2 out]
            n1752 = property on="额定容量" class="DigNum (严格)"("Disabled"=w2301) -> ()  [unwired: 2 in, 2 out]
            n1753 = property on="实际容量" class="DigNum (严格)"("Disabled"=w2301) -> ()  [unwired: 2 in, 2 out]
            n1754 = Select(t=0, s=w2295, f=1) -> (s? t:f=w2294:i32)
            n1755 = property on="生产日期" class="Str"("DisabledEnum"=w2289) -> ()  [unwired: 2 in, 2 out]
            n1756 = property on="电池包序号" class="DigNum (严格)"("DisabledEnum"=w2289) -> ()  [unwired: 2 in, 2 out]
            n1757 = property on="车牌号" class="Str"("DisabledEnum"=w2289) -> ()  [unwired: 2 in, 2 out]
            n1758 = property on="电池包组号" class="DigNum (严格)"("DisabledEnum"=w2289) -> ()  [unwired: 2 in, 2 out]
            n1759 = property on="电池组信息" class="Clust (严格)"("Disabled"=w2294) -> ()  [unwired: 2 in, 2 out]
            n1760 = property on="额定总压" class="DigNum (严格)"("Disabled"=2) -> ()  [unwired: 2 in, 2 out]
            n1761 = property on="产权标识" class="DigNum (严格)"("Disabled"=w2299) -> ()  [unwired: 2 in, 2 out]
            n1762 = property on="应用车型" class="DigNum (严格)"("Disabled"=w2299) -> ()  [unwired: 2 in, 2 out]
            n1763 = property on="放空次数" class="DigNum (严格)"("DisabledEnum"=w2288) -> ()  [unwired: 2 in, 2 out]
            n1764 = property on="充满次数" class="DigNum (严格)"("DisabledEnum"=w2288) -> ()  [unwired: 2 in, 2 out]
            n1765 = property on="充电次数" class="DigNum (严格)"("DisabledEnum"=w2288) -> ()  [unwired: 2 in, 2 out]
            n1766 = property on="最大允许单体电压" class="DigNum (严格)"("Disabled"=w2298) -> ()  [unwired: 2 in, 2 out]
            n1767 = property on="最大允许总电压" class="DigNum (严格)"("Disabled"=w2298) -> ()  [unwired: 2 in, 2 out]
            n1768 = property on="最大允许温度" class="DigNum (严格)"("Disabled"=w2298) -> ()  [unwired: 2 in, 2 out]
            n1769 = property on="最小允许温度" class="DigNum (严格)"("Disabled"=w2298) -> ()  [unwired: 2 in, 2 out]
            n1770 = property on="最大允许充电电流" class="DigNum (严格)"("Disabled"=w2298) -> ()  [unwired: 2 in, 2 out]
            n1771 = property on="最小允许充电电流" class="DigNum (严格)"("Disabled"=w2298) -> ()  [unwired: 2 in, 2 out]
            n1772 = property on="最小允许单体电压" class="DigNum (严格)"("Disabled"=w2298) -> ()  [unwired: 2 in, 2 out]
            n1773 = property on="电流步长" class="DigNum (严格)"("Disabled"=w2298) -> ()  [unwired: 2 in, 2 out]
            n1774 = property on="SOC" class="DigNum (严格)"("Disabled"=w2298) -> ()  [unwired: 2 in, 2 out]
            n1775 = property on="充电总安时" class="DigNum (严格)"("Disabled"=w2294) -> ()  [unwired: 2 in, 2 out]
            n1776 = property on="放电总安时" class="DigNum (严格)"("Disabled"=w2294) -> ()  [unwired: 2 in, 2 out]
            n1777 = Not(x=w2287) -> (.not. x?=w2302:bool)
            n1778 = global read "功能码全局.vi" "24"() -> (w2292:bool[])
            n1779 = global read "功能码全局.vi" "23"() -> (w2293:bool[])
            n1780 = Index Array(array=w2292) -> (element #7=w2290:bool)  [unwired: 8 in, 7 out]
            n1781 = Index Array(array=w2293) -> (element #7=w2291:bool)  [unwired: 8 in, 7 out]
          }
          frame "充电次数" {
            w2307 = 2
            w2316 = 2
            w2317 = 2
            w2308 = 2
            w2318 = 2
            w2304 = FALSE ("1 6")
            n1782 = property on="串联数" class="DigNum (严格)"("Disabled"=w2318) -> ()  [unwired: 2 in, 2 out]
            n1783 = property on="并联数" class="DigNum (严格)"("Disabled"=w2318) -> ()  [unwired: 2 in, 2 out]
            n1784 = property on="电池厂家" class="DigNum (严格)"("Disabled"=w2318) -> ()  [unwired: 2 in, 2 out]
            n1785 = property on="电池类型" class="DigNum (严格)"("Disabled"=w2318) -> ()  [unwired: 2 in, 2 out]
            n1786 = property on="额定能量" class="DigNum (严格)"("Disabled"=w2318) -> ()  [unwired: 2 in, 2 out]
            n1787 = property on="额定容量" class="DigNum (严格)"("Disabled"=w2318) -> ()  [unwired: 2 in, 2 out]
            n1788 = property on="实际容量" class="DigNum (严格)"("Disabled"=w2318) -> ()  [unwired: 2 in, 2 out]
            n1789 = Select(t=0, s=w2313, f=1) -> (s? t:f=w2305:i32)
            n1790 = property on="生产日期" class="Str"("DisabledEnum"=w2307) -> ()  [unwired: 2 in, 2 out]
            n1791 = property on="电池包序号" class="DigNum (严格)"("DisabledEnum"=w2307) -> ()  [unwired: 2 in, 2 out]
            n1792 = property on="车牌号" class="Str"("DisabledEnum"=w2307) -> ()  [unwired: 2 in, 2 out]
            n1793 = property on="电池组信息" class="Clust (严格)"("Disabled"=w2305) -> ()  [unwired: 2 in, 2 out]
            n1794 = property on="电池包组号" class="DigNum (严格)"("DisabledEnum"=w2307) -> ()  [unwired: 2 in, 2 out]
            n1795 = property on="额定总压" class="DigNum (严格)"("Disabled"=w2308) -> ()  [unwired: 2 in, 2 out]
            n1796 = property on="产权标识" class="DigNum (严格)"("Disabled"=w2308) -> ()  [unwired: 2 in, 2 out]
            n1797 = property on="应用车型" class="DigNum (严格)"("Disabled"=w2308) -> ()  [unwired: 2 in, 2 out]
            n1798 = property on="放空次数" class="DigNum (严格)"("DisabledEnum"=w2305) -> (error out=w2306:errorcluster)  [unwired: 2 in, 1 out]
            n1799 = property on="充满次数" class="DigNum (严格)"("DisabledEnum"=w2305) -> ()  [unwired: 2 in, 2 out]
            n1800 = property on="充电次数" class="DigNum (严格)"("DisabledEnum"=w2305) -> ()  [unwired: 2 in, 2 out]
            n1801 = property on="最大允许单体电压" class="DigNum (严格)"("Disabled"=w2317) -> ()  [unwired: 2 in, 2 out]
            n1802 = property on="最大允许总电压" class="DigNum (严格)"("Disabled"=w2317) -> ()  [unwired: 2 in, 2 out]
            n1803 = property on="最大允许温度" class="DigNum (严格)"("Disabled"=w2317) -> ()  [unwired: 2 in, 2 out]
            n1804 = property on="最小允许温度" class="DigNum (严格)"("Disabled"=w2317) -> ()  [unwired: 2 in, 2 out]
            n1805 = property on="最大允许充电电流" class="DigNum (严格)"("Disabled"=w2317) -> ()  [unwired: 2 in, 2 out]
            n1806 = property on="最小允许充电电流" class="DigNum (严格)"(error in=w2306, "Disabled"=w2317) -> ()  [unwired: 1 in, 2 out]
            n1807 = property on="最小允许单体电压" class="DigNum (严格)"("Disabled"=w2317) -> ()  [unwired: 2 in, 2 out]
            n1808 = property on="电流步长" class="DigNum (严格)"("Disabled"=w2317) -> ()  [unwired: 2 in, 2 out]
            n1809 = property on="SOC" class="DigNum (严格)"("Disabled"=w2317) -> ()  [unwired: 2 in, 2 out]
            n1810 = property on="充电总安时" class="DigNum (严格)"("Disabled"=w2316) -> ()  [unwired: 2 in, 2 out]
            n1811 = property on="放电总安时" class="DigNum (严格)"("Disabled"=w2316) -> ()  [unwired: 2 in, 2 out]
            n1812 = Not(x=w2304) -> (.not. x?=w2319:bool)
            n1813 = global read "功能码全局.vi" "24"() -> (w2311:bool[])
            n1814 = global read "功能码全局.vi" "23"() -> (w2312:bool[])
            n1815 = Index Array(array=w2311) -> (element #8=w2310:bool)  [unwired: 8 in, 7 out]
            n1816 = Index Array(array=w2312) -> (element #8=w2309:bool)  [unwired: 8 in, 7 out]
          }
          frame "SOC" {
            w2323 = 2
            w2322 = 2
            w2332 = 2
            w2333 = 2
            w2334 = 2
            w2336 = 2
            w2321 = FALSE ("1 6")
            n1817 = property on="串联数" class="DigNum (严格)"("Disabled"=w2336) -> ()  [unwired: 2 in, 2 out]
            n1818 = property on="并联数" class="DigNum (严格)"("Disabled"=w2336) -> ()  [unwired: 2 in, 2 out]
            n1819 = property on="电池厂家" class="DigNum (严格)"("Disabled"=w2336) -> ()  [unwired: 2 in, 2 out]
            n1820 = property on="电池类型" class="DigNum (严格)"("Disabled"=w2336) -> ()  [unwired: 2 in, 2 out]
            n1821 = property on="额定能量" class="DigNum (严格)"("Disabled"=w2336) -> ()  [unwired: 2 in, 2 out]
            n1822 = property on="额定容量" class="DigNum (严格)"("Disabled"=w2336) -> ()  [unwired: 2 in, 2 out]
            n1823 = property on="实际容量" class="DigNum (严格)"("Disabled"=w2336) -> ()  [unwired: 2 in, 2 out]
            n1824 = Select(t=0, s=w2329, f=1) -> (s? t:f=w2328:i32)
            n1825 = property on="生产日期" class="Str"("DisabledEnum"=w2323) -> ()  [unwired: 2 in, 2 out]
            n1826 = property on="电池包序号" class="DigNum (严格)"("DisabledEnum"=w2323) -> ()  [unwired: 2 in, 2 out]
            n1827 = property on="车牌号" class="Str"("DisabledEnum"=w2323) -> ()  [unwired: 2 in, 2 out]
            n1828 = property on="电池包组号" class="DigNum (严格)"("DisabledEnum"=w2323) -> ()  [unwired: 2 in, 2 out]
            n1829 = property on="电池组信息" class="Clust (严格)"("Disabled"=w2328) -> ()  [unwired: 2 in, 2 out]
            n1830 = property on="SOC" class="DigNum (严格)"("Disabled"=w2328) -> ()  [unwired: 2 in, 2 out]
            n1831 = property on="额定总压" class="DigNum (严格)"("Disabled"=2) -> ()  [unwired: 2 in, 2 out]
            n1832 = property on="产权标识" class="DigNum (严格)"("Disabled"=w2334) -> ()  [unwired: 2 in, 2 out]
            n1833 = property on="应用车型" class="DigNum (严格)"("Disabled"=w2334) -> ()  [unwired: 2 in, 2 out]
            n1834 = property on="放空次数" class="DigNum (严格)"("DisabledEnum"=w2322) -> ()  [unwired: 2 in, 2 out]
            n1835 = property on="充满次数" class="DigNum (严格)"("DisabledEnum"=w2322) -> ()  [unwired: 2 in, 2 out]
